vi "Send Request.vi"(0 "IPEndPoint":T2, 7 "TCPMessage":T1, 9 "timeout ms (25000)":i32=5000, 11 "error in (no error)":errorcluster) -> (4 "IPEndPoint thru":T2, 8 "Response":T1, 15 "error out":errorcluster)   [LabVIEW 2020, in "epl-network.lvlib"]
uses:
  epl-network.lvlib
  Typedefs/TCP Message.ctl
  Typedefs/IPEndPoint.ctl
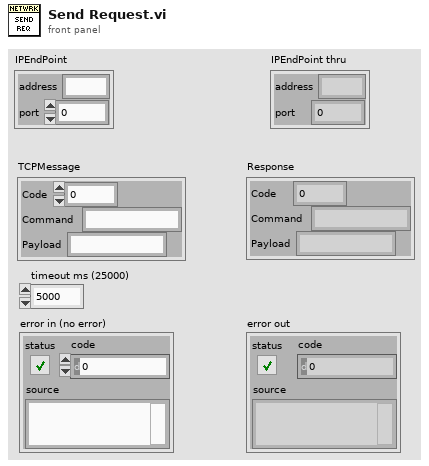
[diagram p1: front panel]
types:
  T1 = typedef "epl-network.lvlib/TCP Message.ctl" = cluster{"Code":i32, "Command":string, "Payload":string}
  T2 = typedef "epl-network.lvlib/IPEndPoint.ctl" = cluster{"address":string, "port":i32}
  T3 = enum16{"big-endian, network order", "native, host order", "little-endian"}
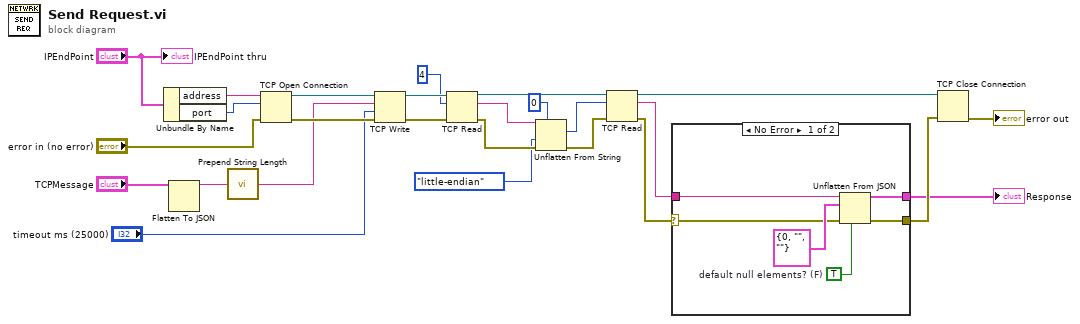
[diagram p0: block diagram]
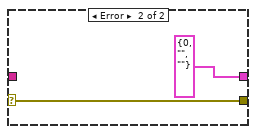
[diagram p2: hidden frame]
diagram:
  n1 = Unbundle By Name("IPEndPoint") -> ("address"=w25:string, "port"=w24:i32)
  n2 = Flatten To JSON(anything="TCPMessage") -> (JSON string=w18:string)  [unwired: 2 in, 1 out]
  n3 = call "Prepend String Length.vi"("String"=w18) -> ("Length-prefixed string"=w17:string)  [unwired: 14 in]
  n4 = TCP Open Connection(address=w25, remote port or service name=w24, error in (no error)="error in (no error)") -> (connection ID=w22:refnum<k5>, error out=w20:errorcluster)  [unwired: 2 in]
  n5 = TCP Write(connection ID=w22, data in=w17, error in (no error)=w20, 9:"timeout ms (25000)") -> (connection ID out=w16:refnum<k5>, error out=w15:errorcluster)  [unwired: 1 out]
  n6 = TCP Read(connection ID=w16, bytes to read=4, error in (no error)=w15) -> (connection ID out=w9:refnum<k5>, data out=w4:string, error out=w8:errorcluster)  [unwired: 2 in]
  n7 = Unflatten From String(type=0, binary string=w4, byte order (0:big-endian, network order)=T3."little-endian", error in (no error)=w8) -> (value=w11:i32, error out=w10:errorcluster)  [unwired: 1 in, 1 out]
  n8 = TCP Read(connection ID=w9, bytes to read=w11, error in (no error)=w10) -> (connection ID out=w14:refnum<k5>, data out=w3:string, error out=w2:errorcluster)  [unwired: 2 in]
  n9 = case shown="No Error" w2 {
    selector: w2 -> [w28 w33]
    tunnel: [w32 w33] -> w13
    tunnel: [w31 T1 {"Code"=0, "Command"="", "Payload"=""} ("Response")] -> w5
    tunnel: w3 -> [w30 _]
    frame No Error {
      w27 = TRUE  # default null elements? (F)
      n10 = Unflatten From JSON(JSON string=w30, type and defaults=T1 {"Code"=0, "Command"="", "Payload"=""} ("Response"), default null elements? (F)=w27, error in (no error)=w28) -> (value=w31:T1, error out=w32:errorcluster)  [unwired: 3 in]
    }
    frame Error {
    }
  }
  "Response" <- w5
  n11 = TCP Close Connection(connection ID=w14, error in (no error)=w13) -> (error out=→"error out":errorcluster)  [unwired: 1 in, 1 out]
  "IPEndPoint thru" <- "IPEndPoint"
